vi "Actor Core.vi"(8 "error in":errorcluster, 11 "Sample Error Reporter in":refnum<class "Sample Error Reporter.lvclass">) -> (0 "error out":errorcluster, 3 "Actor out":refnum<class "Actor.lvclass">)   [LabVIEW 2024, in "Sample Error Reporter.lvlib" / "Sample Error Reporter.lvclass"]
doc: "<p>(<strong>Filename</strong>: <span class=\"dnl\">Actor Framework.lvlib:Actor.lvclass:Actor Core.vi</span>)</p>\n<p>Receives messages to the actor, reacts to them, and initiates any error handling that may shut the actor down.</p>\n<p>Descendant classes may override this VI to append parallel tasks for the actor to complete while it handles messages. Overrides use the <a href=\"nihelplauncher://docs/csh?context=lvcore_glang_udclass\">Call Parent Class Method</a> node.</p>"
uses:
  Sample Error Reporter.lvclass
  <vilib>/ActorFramework/Actor/Actor.lvclass
  <vilib>/ActorFramework/Actor/Actor.lvclass/Actor.ctl
  <vilib>/ActorFramework/Message Enqueuer/Message Enqueuer.lvclass/Message Enqueuer.ctl
  Sample Error Reporter.lvclass/Sample Error Reporter.ctl
  <vilib>/ActorFramework/Message Enqueuer/Init from Existing Queue.vi
  <vilib>/ActorFramework/Message Enqueuer/Enqueue.vi
  Sample Error Reporter Messages/Generate Error Msg/Generate Error Msg.lvclass
  <vilib>/ActorFramework/Stop Msg/Stop Msg.lvclass
  <vilib>/ActorFramework/Message Priority Queue/Priority Enqueue.vi
  src/Error Reporting Actor/Error Reporter/Error Reporter/Error Reporter.lvclass
  <vilib>/ActorFramework/Message Enqueuer/Message Enqueuer.lvclass
panel:
  in  "Generate Error":bool
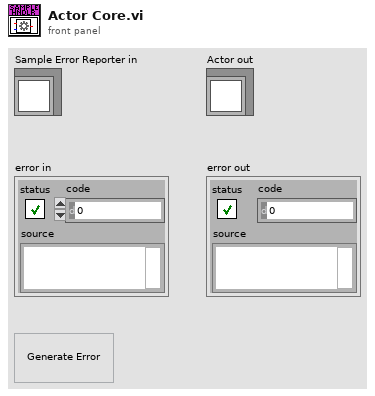
[diagram p1: front panel]
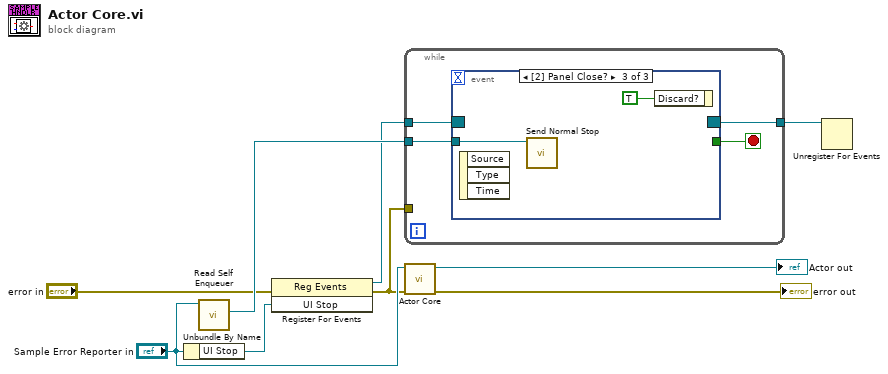
[diagram p0: block diagram]
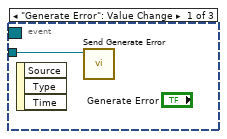
[diagram p2: hidden frame]
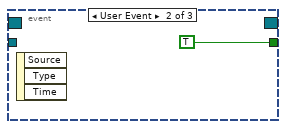
[diagram p3: hidden frame]
diagram:
  n1 = Unbundle By Name("Sample Error Reporter in") -> ("UI Stop"=w5:refnum<user-event>)
  n2 = call <vilib>:"Read Self Enqueuer.vi"("Actor"="Sample Error Reporter in") -> ("Self Enqueuer"=w7:refnum<class "Message Enqueuer.lvclass">)  [unwired: 10 in]
  n3 = register-events(error in="error in", w5) -> (reference out=w4:refnum<event-registration>, error out=w2:errorcluster)  [unwired: 1 in]
  n4 = while {
    tunnel: w7 -> [w13]
    tunnel: w4 -> [w12]
    tunnel: w2 -> [_]
    tunnel: [w10] -> w1
    stop <- w11 stop-if-true
    n5 = event shown="[2] Panel Close?" {
      selector: w12 -> [_ _ _]
      dyn-events: [_ _ _] -> w10
      timeout: _ -> [_ _ _]
      tunnel: w13 -> [w14 _ w16]
      tunnel: [_ TRUE _] -> w11
      event "Generate Error": Value Change {
        n6 = event-data() -> ()  [unwired: 1 in, 3 out]
        n7 = call "Send Generate Error.vi"("Message Enqueuer"=w14) -> ()  [unwired: 9 in, 2 out]
      }
      event User Event {
        n8 = event-data() -> ()  [unwired: 1 in, 3 out]
      }
      event Panel Close? {
        n9 = event-data() -> ()  [unwired: 1 in, 3 out]
        n10 = call <vilib>:"Send Normal Stop.vi"("Message Enqueuer"=w16) -> ()  [unwired: 10 in, 1 out]
        n11 = event-data("Discard?"=TRUE) -> ()  [unwired: 1 in, 1 out]
      }
    }
  }
  n12 = call-parent "Actor Core.vi"("error in"=w2, "Actor in"="Sample Error Reporter in") -> ("error out"=→"error out":errorcluster, "Actor out"=→"Actor out":refnum<class "Actor.lvclass">)  [unwired: 8 in]
  n13 = Unregister For Events(event registration refnum=w1) -> ()  [unwired: 1 in, 1 out]
